vi "Revision Query Core.vi"(8 "error in (no error)":errorcluster, 11 "BNT_ULx-MCSV-Ctr2Freq in":refnum<class "BNT_ULx-MCSV-Ctr2Freq.lvclass">) -> (0 "error out":errorcluster, 1 "Firmware Revision":string, 2 "Driver Revision":string, 3 "BNT_ULx-MCSV-Ctr2Freq out":refnum<class "BNT_ULx-MCSV-Ctr2Freq.lvclass">)   [LabVIEW 2021, in "BNT_ULx.lvlib" / "BNT_ULx-MCSV-Ctr2Freq.lvclass"]
uses:
  BNT_ULx-MCSV-Ctr2Freq.lvclass
  BNT_ULx-MCSV/BNT_ULx-MCSV.lvclass
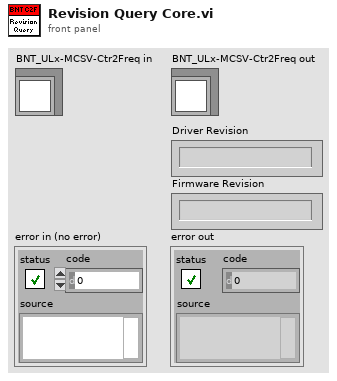
[diagram p1: front panel]
types:
  T1 = cluster{"Major":u16, "Minor":u16, "Fix":u16, "Build":u16}
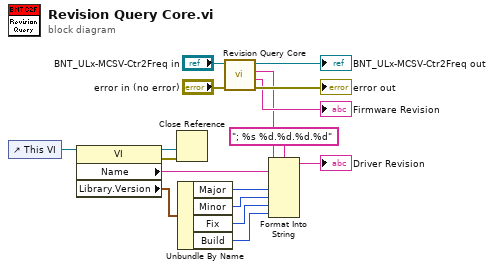
[diagram p0: block diagram]
diagram:
  n1 = control-ref of="This VI"() -> (w12:refnum<vi>)
  n2 = property class="VI"(reference=w12) -> (reference out=w10:refnum<vi>, error out=w11:errorcluster, "Name"=w3:string, "Library.Version"=w9:T1)  [unwired: 1 in]
  n3 = Close Reference(reference=w10, error in (no error)=w11) -> ()  [unwired: 1 out]
  n4 = Unbundle By Name(w9) -> ("Major"=w7:u16, "Minor"=w6:u16, "Fix"=w5:u16, "Build"=w4:u16)
  n5 = call-parent "Revision Query Core.vi"("error in (no error)"="error in (no error)", "BNT_ULx-MCSV in"="BNT_ULx-MCSV-Ctr2Freq in") -> ("error out"=→"error out":errorcluster, "Firmware Revision"=→"Firmware Revision":string, "Driver Revision"=w2:string, "BNT_ULx-MCSV out"=→"BNT_ULx-MCSV-Ctr2Freq out":refnum<class "BNT_ULx-MCSV-Ctr2Freq.lvclass">)  [unwired: 6 in]
  n6 = Format Into String(format string="; %s %d.%d.%d.%d" ("Driver Revision"), initial string=w2, w3, w7, w6, w5, w4) -> (resulting string=→"Driver Revision":string)  [unwired: 1 in, 1 out]
